vi "configureAcquisition.vi"(6 "imagePaths":path[](array[path]), 7 "saveImages?":bool, 8 "error in (no error)":errorcluster, 9 "number of Images":i32, 10 "CameraSettings":refnum<class "CamaraSettings.lvclass">, 11 "WinX32Camera in":refnum<class "WinX32Camera.lvclass">) -> (0 "error out":errorcluster, 3 "WinX32Camera out":refnum<class "WinX32Camera.lvclass">)   [LabVIEW 2011, in "WinX32Camera.lvclass"]
uses:
  WinX32Camera.lvclass
  Tools/CameraSettings/CamaraSettings.lvclass
  WinX32Camera.lvclass/WinX32Camera.ctl
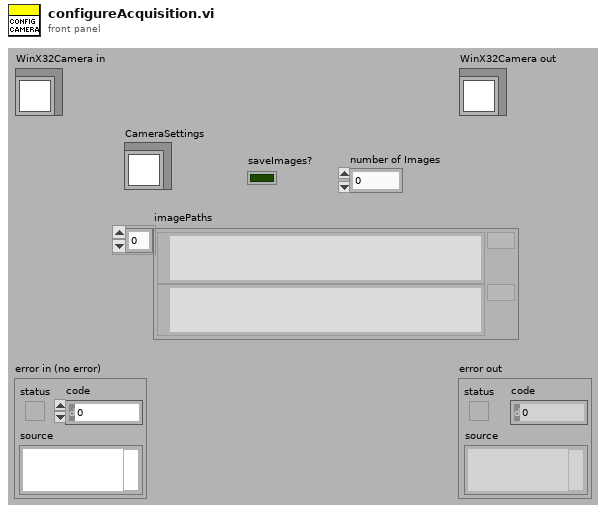
[diagram p1: front panel]
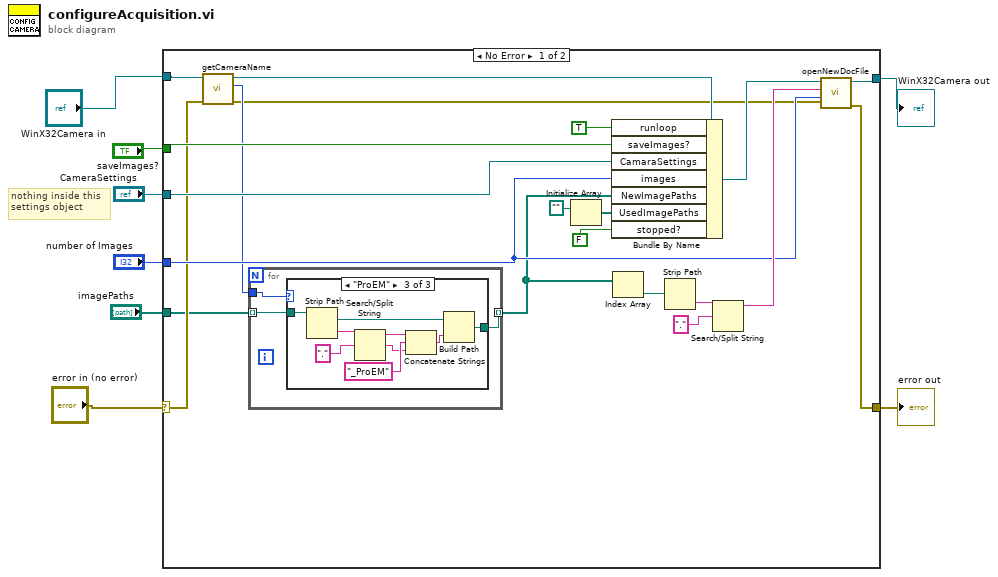
[diagram p0: block diagram]
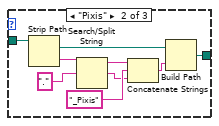
[diagram p3: hidden frame]
diagram:
  # "nothing inside this\nsettings object"
  n1 = case shown="No Error" "error in (no error)" {
    selector: "error in (no error)" -> [w13 w53]
    tunnel: [w18 w53] -> w7
    tunnel: [w19 w52] -> w5
    tunnel: "WinX32Camera in" -> [w15 w52]
    tunnel: "saveImages?" -> [w29 _]
    tunnel: "CameraSettings" -> [w28 _]
    tunnel: "imagePaths" -> [w12 _]
    tunnel: "number of Images" -> [w20 _]
    frame No Error {
      n2 = call "getCameraName.vi"("error in (no error)"=w13, "WinX32Camera in"=w15) -> ("error out"=w9:errorcluster, "Camera"=w10:enum16{"Simulation", "Pixis", "ProEM"}, "WinX32Camera out"=w14:refnum<class "WinX32Camera.lvclass">)  [unwired: 7 in]
      n3 = for {
        tunnel: w12 -> [w31] mode=indexing
        tunnel: [w30] -> w11 mode=indexing
        tunnel: w10 -> [w32]
        n4 = case shown="\"ProEM\"" w32 {
          tunnel: w31 -> [w33 w40 w49]
          tunnel: [w33 w34 w43] -> w30
          frame "Simulation", Default {
          }
          frame "Pixis" {
            n5 = Strip Path(path=w40) -> (stripped path=w35:path, name=w42:string)
            n6 = Search/Split String(string=w42, search string/char (-)=".") -> (substring before match=w39:string, match + rest of string=w37:string)  [unwired: 1 in, 1 out]
            n7 = Concatenate Strings(w39, "_Pixis", w37) -> (w36:string)
            n8 = Build Path(base path=w35, name or relative path=w36) -> (appended path=w34:path)
          }
          frame "ProEM" {
            n9 = Strip Path(path=w49) -> (stripped path=w44:path, name=w51:string)
            n10 = Search/Split String(string=w51, search string/char (-)=".") -> (substring before match=w48:string, match + rest of string=w46:string)  [unwired: 1 in, 1 out]
            n11 = Concatenate Strings(w48, "_ProEM", w46) -> (w45:string)
            n12 = Build Path(base path=w44, name or relative path=w45) -> (appended path=w43:path)
          }
        }
      }
      n13 = Initialize Array(path "") -> (w26:path[])  [unwired: 1 in]
      n14 = Bundle By Name(cluster=w14, "runloop"=TRUE, "saveImages?"=w29, "CamaraSettings"=w28, "images"=w20, "NewImagePaths"=w11, "UsedImagePaths"=w26, "stopped?"=FALSE) -> (w22:refnum<class "WinX32Camera.lvclass">)
      n15 = Index Array(array=w11) -> (element=w25:path)  [unwired: 1 in]
      n16 = Strip Path(path=w25) -> (name=w24:string)  [unwired: 1 out]
      n17 = Search/Split String(string=w24, search string/char (-)=".") -> (substring before match=w21:string)  [unwired: 1 in, 2 out]
      n18 = call "openNewDocFile.vi"("error in (no error)"=w9, "# of images"=w20, "name"=w21, "WinX32Camera in"=w22) -> ("error out"=w18:errorcluster, "WinX32Camera out"=w19:refnum<class "WinX32Camera.lvclass">)  [unwired: 6 in]
    }
    frame Error {
    }
  }
  "error out" <- w7
  "WinX32Camera out" <- w5
